vi "Read Boolean Array.vi"(8 "error in":errorcluster, 11 "Config Data in":refnum<class "Config Data.lvclass">) -> (0 "error out":errorcluster, 2 "Data Out":bool[](array[boolean]), 3 "Config Data out":refnum<class "Config Data.lvclass">)   [LabVIEW 2016, in "Config Data.lvclass"]
uses:
  Config Data.lvclass
  Config Data.lvclass/Config Data.ctl
  <vilib>/Utility/config.llb/Read Key (String).vi
  <vilib>/Utility/config.llb/NI_LVConfig.lvlib
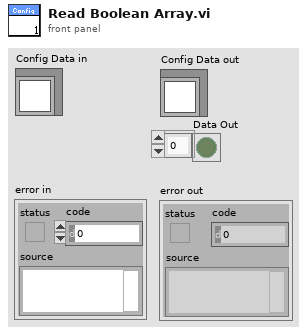
[diagram p1: front panel]
types:
  T1 = typedef "NI_LVConfig.lvlib/Config Data RefNum.ctl" = refnum<k1>
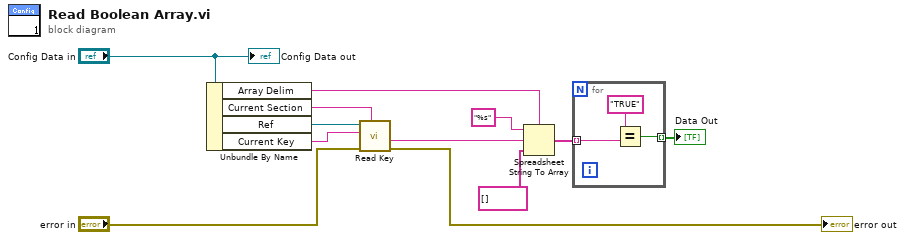
[diagram p0: block diagram]
diagram:
  n1 = Unbundle By Name("Config Data in") -> ("Array Delim"=w1:string, "Current Section"=w8:string, "Ref"=w9:T1, "Current Key"=w7:string)
  n2 = call-poly <vilib>:"Read Key.vi"("section"=w8, "error in (no error)"="error in", "key"=w7, "refnum"=w9) -> ("error out"=→"error out":errorcluster, "value"=w6:string)  [unwired: 4 in, 2 out]
  n3 = Spreadsheet String To Array(delimiter (Tab)=w1, format string="%s", spreadsheet string=w6, array type (2D Dbl)=string[] []) -> (array=w3:string[])
  n4 = for {
    tunnel: w3 -> [w15] mode=indexing
    tunnel: [w13] -> w2 mode=indexing
    n5 = Equal?(x="TRUE", y=w15) -> (x = y?=w13:bool)
  }
  "Data Out" <- w2
  "Config Data out" <- "Config Data in"
